vi "Teleop.vi"(10 "Match Info":T1={"Autonomous Elapsed Seconds"=0.0, "TeleOp Elapsed Seconds"=0.0, "Disabled Elapsed Seconds"=0.0, "Visited Autonomous"=FALSE, "Visited TeleOp"=FALSE, "Visited Disabled"=FALSE, "Autonomous Settings"={"Autonomous Style"=enum."Independent", "VI Refnum"=refnum}}, 11 "Call Context":T2) -> ()   [LabVIEW 2011]
doc: "This VI is called for each TeleOp packet received from the DS where the robot is not disabled. It is often used to read from the joysticks and update I/O or to update setpoints for timed control loops. It should complete and return within 20 milliseconds or it may miss DS packets."
uses:
  <vilib>/Rock Robotics/WPI/DriverStation/WPI_DriverStationDerivedRobotMode.ctl
  <vilib>/Rock Robotics/WPI/DriverStation/WPI_DriverStationMatch Info.ctl
  TypeDefs/Dashboard Data TypeDef.ctl
  Robot Global Data.vi
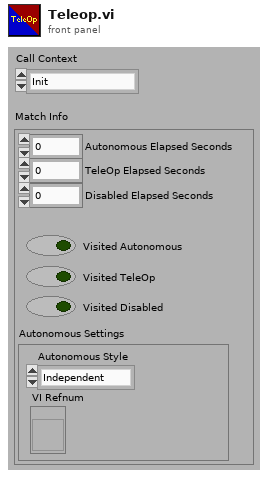
[diagram p1: front panel]
types:
  T1 = typedef "WPI_DriverStationMatch Info.ctl" = cluster{"Autonomous Elapsed Seconds":dbl, "TeleOp Elapsed Seconds":dbl, "Disabled Elapsed Seconds":dbl, "Visited Autonomous":bool, "Visited TeleOp":bool, "Visited Disabled":bool, "Autonomous Settings":cluster{"Autonomous Style":enum16{"Iterative", "Independent"}, "VI Refnum":refnum<vi>}}
  T2 = typedef "WPI_DriverStationDerivedRobotMode.ctl" = enum16{"Init", "Execute", "Stop"}
  T3 = typedef "Dashboard Data TypeDef.ctl" = cluster{"Number of Balls":i32, "Shooting Manual Override?":bool, "Bridge Mode?":bool, "Shooter":bool, "Shooter At Speed?":bool, "Aligning Mode?":bool}
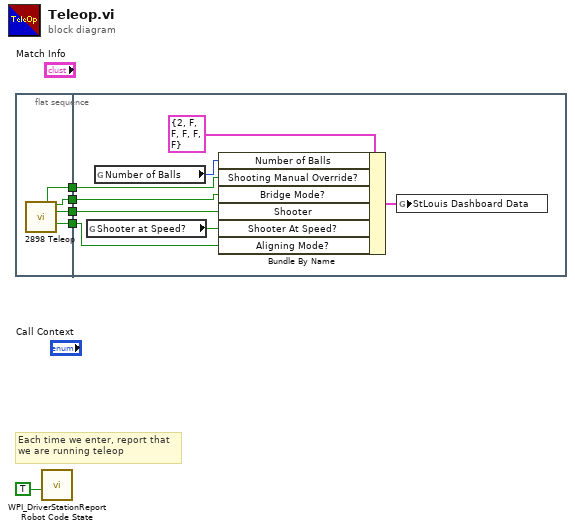
[diagram p0: block diagram]
diagram:
  # "Each time we enter, report that\nwe are running teleop"
  n1 = flat-sequence {
    tunnel: [w9] -> w4
    tunnel: [w8] -> w3
    tunnel: [w7] -> w2
    tunnel: [w6] -> w1
    tunnel: w4 -> [w15]
    tunnel: w3 -> [w16]
    tunnel: w2 -> [w17]
    tunnel: w1 -> [w12]
    frame #0 {
      n2 = call "2898 Teleop.vi"() -> ("Shooting Manual Override?"=w7:bool, "Bridge Mode?"=w8:bool, "Shooter Is Front"=w9:bool, "Aligning Mode?"=w6:bool)  [unwired: 12 in]
    }
    frame #1 {
      n3 = global read "Robot Global Data.vi" "Shooter at Speed?"() -> (w14:bool)
      n4 = global read "Robot Global Data.vi" "Number of Balls"() -> (w10:i32)
      n5 = Bundle By Name(cluster=T3 {"Number of Balls"=2, "Shooting Manual Override?"=FALSE, "Bridge Mode?"=FALSE, "Shooter"=FALSE, "Shooter At Speed?"=FALSE, "Aligning Mode?"=FALSE} ("Cluster"), "Number of Balls"=w10, "Shooting Manual Override?"=w17, "Bridge Mode?"=w16, "Shooter"=w15, "Shooter At Speed?"=w14, "Aligning Mode?"=w12) -> (w11:T3)
      n6 = global write "Robot Global Data.vi" "StLouis Dashboard Data"(w11) -> ()
    }
  }
  n7 = call <vilib>:"WPI_DriverStationReport Robot Code State.vi"("TeleOp"=TRUE ("Autonomous")) -> ()  [unwired: 10 in, 1 out]
